vi "JSON validation example.vi"() -> ()   [LabVIEW 2015]
uses:
  <vilib>/addons/_JKI.lib/Serialization/JSON/JKI JSON Serialization.lvlib
panel:
  out "Element name":string
  in  "Comparing JSON":string
  in  "Reference JSON":string
  out "error out":errorcluster
  in  "error in (no error)":errorcluster
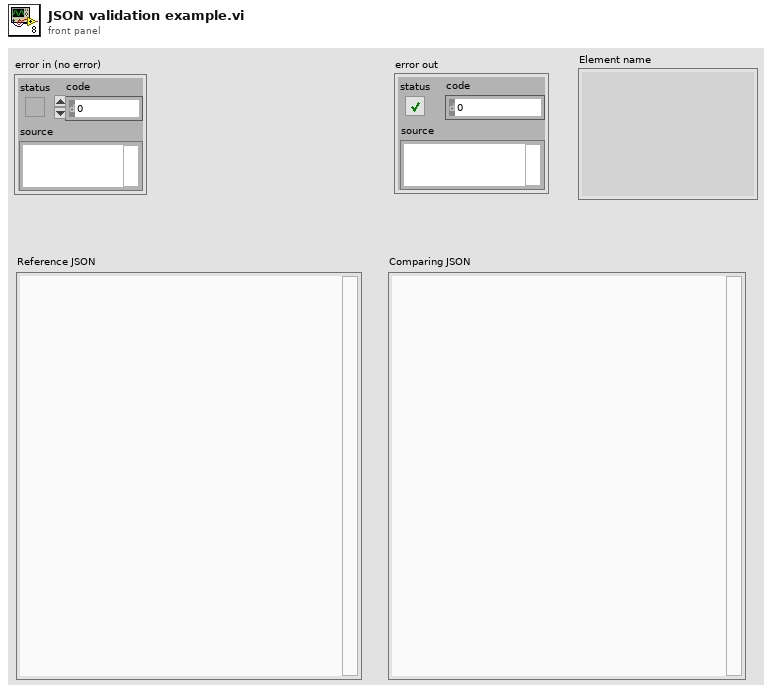
[diagram p1: front panel]
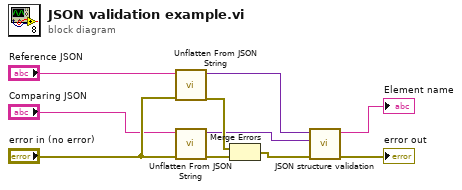
[diagram p0: block diagram]
diagram:
  n1 = call <vilib>:"Unflatten From JSON String.vi"("error in (no error)"="error in (no error)", "JSON String"="Reference JSON") -> ("error out"=w7:errorcluster, "Variant"=w3:variant)  [unwired: 8 in]
  n2 = call <vilib>:"Unflatten From JSON String.vi"("error in (no error)"="error in (no error)", "JSON String"="Comparing JSON") -> ("error out"=w8:errorcluster, "Variant"=w2:variant)  [unwired: 8 in]
  n3 = Merge Errors(w7, w8) -> (w6:errorcluster)
  n4 = call "JSON structure validation.vi"("error in (no error)"=w6, "Compare\nvariant"=w2, "Reference\nvariant"=w3) -> ("error out"=→"error out":errorcluster, "Element name"=→"Element name":string)  [unwired: 6 in, 1 out]
